vi "Get Continuous Data from Com Port in LabView.vi"() -> ()   [LabVIEW 2014]
doc: "This example performs writes and reads on a serial port, as directed by the user. You can press the Write and Read buttons, and change the Read Count, while the example is running.\n\nThe parameters set for the serial port must match the parameters of the connected instrument or device. In this example, the Read Count parameter specifies the number of bytes that the serial port reads. If there were more bytes at the port than the specified number, those bytes would not be read. If there were less bytes at the port than the specified number, you would receive a timeout error.\n\nThis example expands upon the flow control options for XON and XOFF, allowing the user to choose those control characters. Also, the user can enable or disable a termination character. Some devices require a termination character in order to identify the end of command strings. Some devices send a termination character to signify the end of data to be read. This example shows how you can end the Read operation once a termination character is detected in the buffer and/or append a termination character at the end of the Write data."
uses:
  <vilib>/Instr/_visa.llb/VISA Configure Serial Port (Instr).vi
panel:
  out "Data 1D":dbl[](array[numeric]) caption="array" format="%#_2f"
  in  "Stop":bool
  in  "Read Count":u32=1000
  out "Response":string
  in  "Start Reading":bool
  in  "VISA resource name":refnum<visa-resource-name>="COM1"
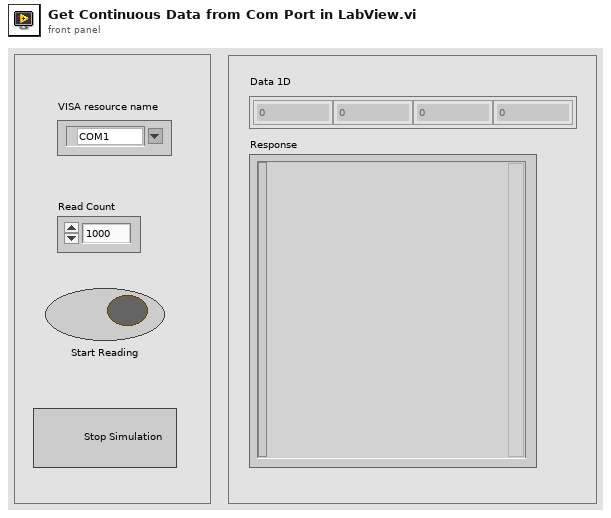
[diagram p1: front panel]
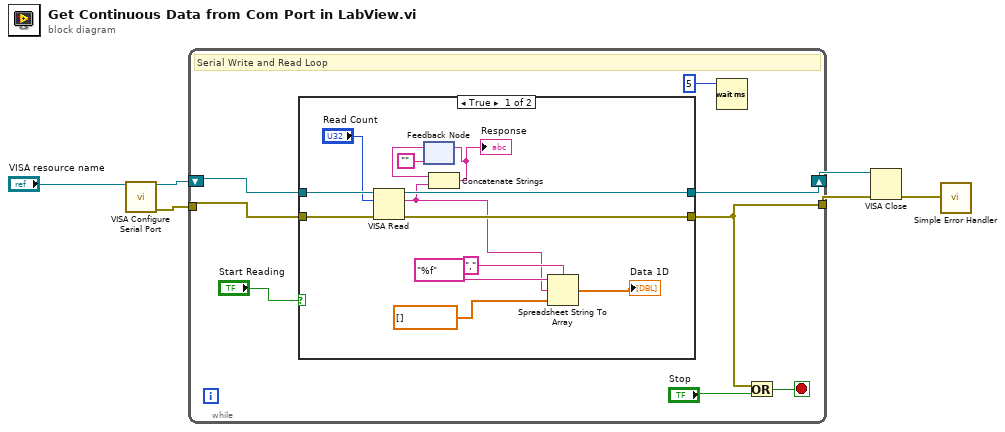
[diagram p0: block diagram]
diagram:
  n1 = call-poly "VISA Configure Serial Port"("VISA resource name"="VISA resource name") -> ("VISA resource name out"=w2:refnum<visa-resource-name>, "error out"=w1:errorcluster)  [unwired: 9 in, 4 out]
  n2 = while {
    shift-right: [w14] -> w3
    shift-left: w2 -> [w11]
    tunnel: w1 -> [w10]
    tunnel: [w12] -> w4
    stop <- w7 stop-if-true
    # "Serial Write and Read Loop"
    n3 = case shown="True" "Start Reading" {
      tunnel: [w25 w29] -> w14
      tunnel: w11 -> [w27 w29]
      tunnel: [w23 w28] -> w12
      tunnel: w10 -> [w26 w28]
      frame True {
        n4 = VISA Read(VISA resource name=w27, byte count="Read Count", error in (no error)=w26) -> (VISA resource name out=w25:refnum<visa-resource-name>, read buffer=w16:string, error out=w23:errorcluster)  [unwired: 1 out]
        n5 = feedback #1("") -> (w22:string)
        n6 = Concatenate Strings(w22, w16) -> (w17:string)
        "Response" <- w17
        n7 = feedback-in #1(w17) -> ()
        n8 = Spreadsheet String To Array(delimiter (Tab)=",", format string="%f", spreadsheet string=w16, array type (2D Dbl)=dbl[] [] ("Data Graph")) -> (array=→"Data 1D":dbl[])
      }
      frame False {
      }
    }
    n9 = Wait (ms)(milliseconds to wait=u32 5) -> ()  [unwired: 1 out]
    n10 = Or(x=w12, y="Stop") -> (x .or. y?=w7:bool)
  }
  n11 = VISA Close(VISA resource name=w3, error in (no error)=w4) -> (error out=w5:errorcluster)
  n12 = call <vilib>:"Simple Error Handler.vi"("error in (no error)"=w5) -> ()  [unwired: 1 in, 8 out]
